vi "tokenize_string.vi"(8 "error in (no error)":errorcluster, 10 "delimiter":string, 11 "input_string":string) -> (0 "error out":errorcluster, 1 "last":string, 2 "first":string, 3 "delimited_string []":string[](array[string]))   [LabVIEW 2015, in "lv-dropbox.lvlib"]
uses:
  lv-dropbox.lvlib
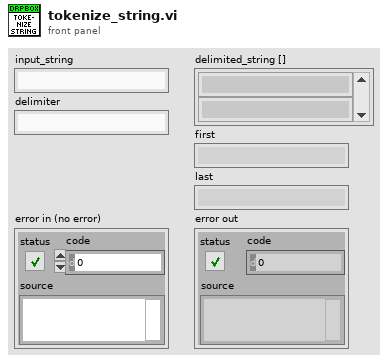
[diagram p1: front panel]
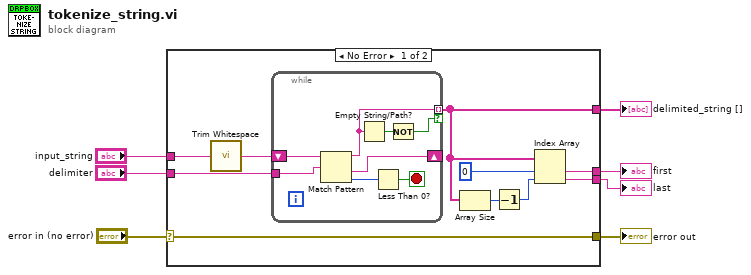
[diagram p0: block diagram]
diagram:
  n1 = case shown="No Error" "error in (no error)" {
    selector: "error in (no error)" -> [w15 w26]
    tunnel: "delimiter" -> [w17 _]
    tunnel: [w13 _] -> w6
    tunnel: "input_string" -> [w16 _]
    tunnel: [w15 w26] -> w3
    tunnel: [w10 _] -> w2
    tunnel: [w9 _] -> w1
    frame No Error {
      n2 = call <vilib>:"Trim Whitespace.vi"("string"=w16) -> ("trimmed string"=w8:string)  [unwired: 1 in]
      n3 = while {
        shift-right: [w24] -> _
        shift-left: w8 -> [w25]
        tunnel: [w20] -> w13 mode=indexing if=w18
        tunnel: w17 -> [w21]
        stop <- w22 stop-if-true
        n4 = Match Pattern(string=w25, regular expression=w21) -> (before substring=w20:string, after substring=w24:string, offset past match=w23:i32)  [unwired: 1 in, 1 out]
        n5 = Empty String/Path?(string/path=w20) -> (empty?=w19:bool)
        n6 = Less Than 0?(x=w23) -> (x < 0?=w22:bool)
        n7 = Not(x=w19) -> (.not. x?=w18:bool)
      }
      n8 = Array Size(array=w13) -> (size(s)=w12:i32)
      n9 = Decrement(x=w12) -> (x-1=w11:i32)
      n10 = Index Array(array=w13, index #1=0 ("index"), index #2=w11) -> (element #1=w10:string, element #2=w9:string)
    }
    frame Error {
    }
  }
  "delimited_string []" <- w6
  "error out" <- w3
  "last" <- w1
  "first" <- w2
